vi "2D barcode scanning no PSD 2 scanners.vi"() -> ()   [LabVIEW 2017]
panel:
  out "Horizontal Mirror Driving Angle 1":dynamicdata(graph)
  out "Horizontal Angle Vs. Photodiode Falling 2":cluster{"X":dbl[], "Y":dbl[]}[](graph) caption="XY Graph"
  out "Horizontal Mirror Angle 2":dbl[](graph)
  out "Horizontal Mirror Driving Angle 2":dynamicdata(graph)
  out "Photodiode 2":dynamicdata(graph)
  out "Photodiode 1":dynamicdata(graph)
  in  "All points":bool
  out "Vertical Mirror Angle":dynamicdata(graph)
  out "Horizontal Mirror Angle 1":dynamicdata(graph)
  out "Vertical Angle vs. Photodiode":cluster{"Y":dbl[], "Y":dbl[]}[](graph)
  out "Horizontal Angle vs. Photodiode Falling  1":cluster{"Y":dbl[], "Y":dbl[]}[](graph)
  out "Horizontal Mirror Driving Voltage (common)":dynamicdata(graph)
  out "Vertical Mirror Driving Voltage":dynamicdata(graph)
  in  "stop (F)":bool
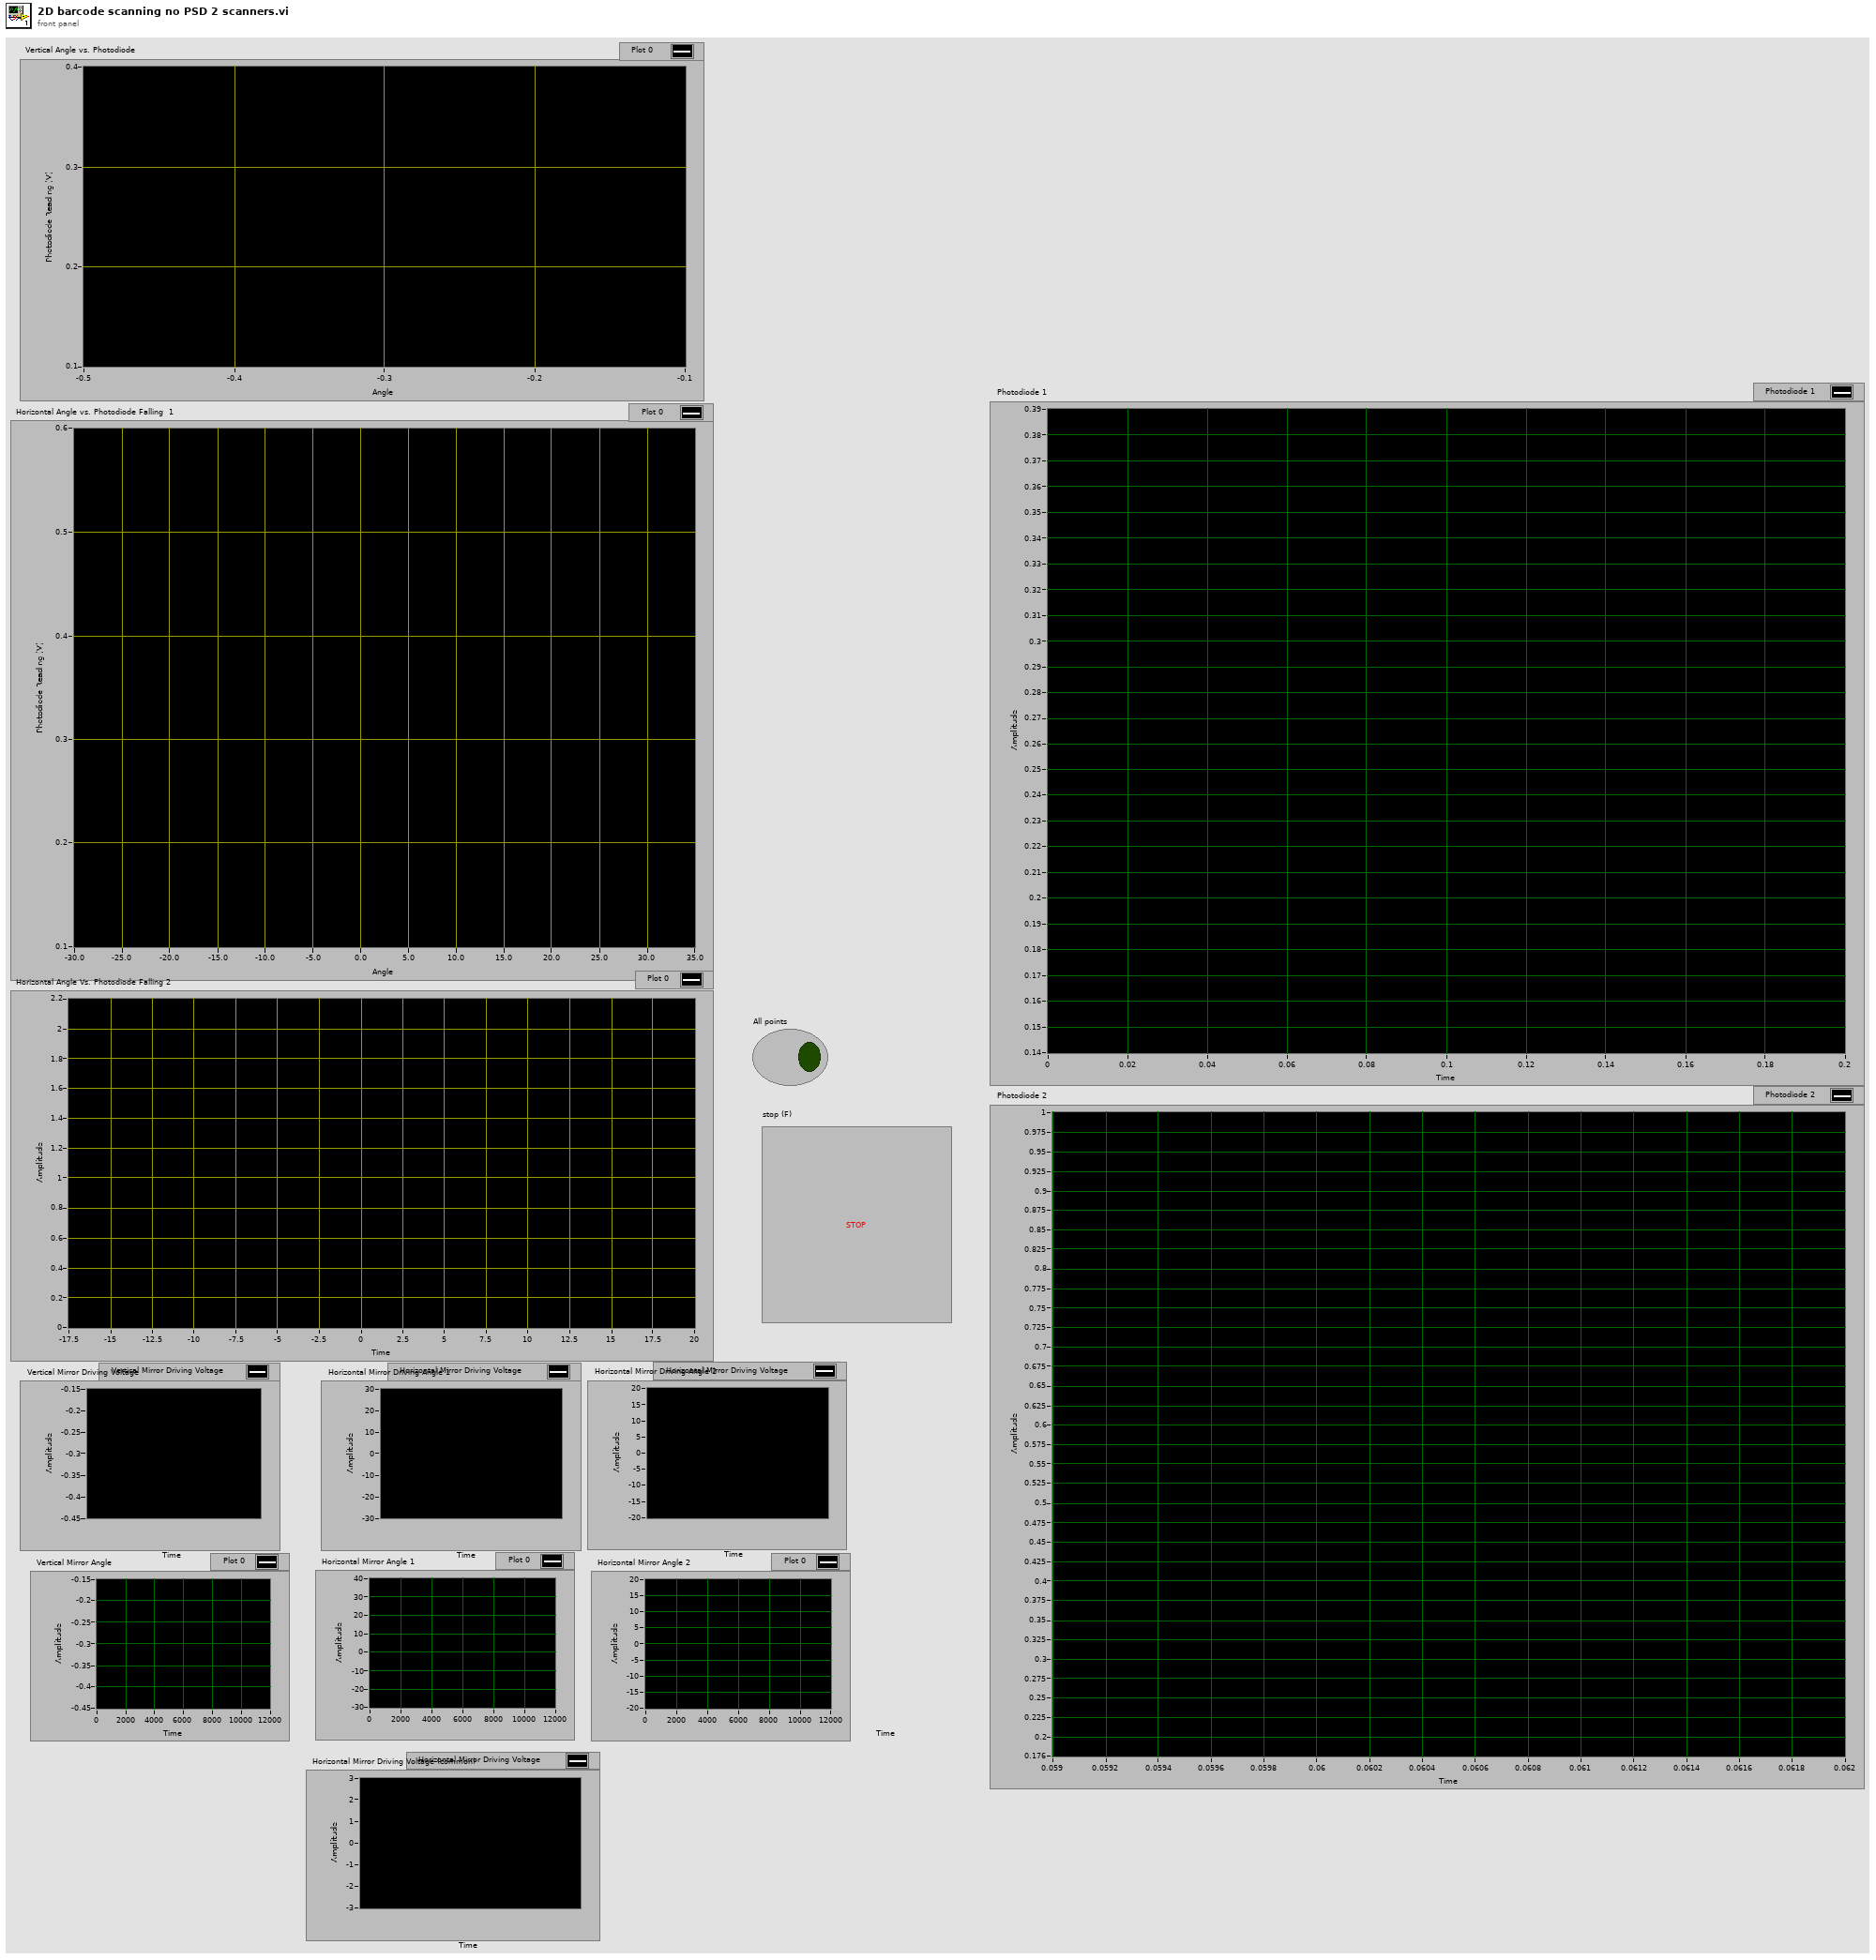
[diagram p1: front panel]
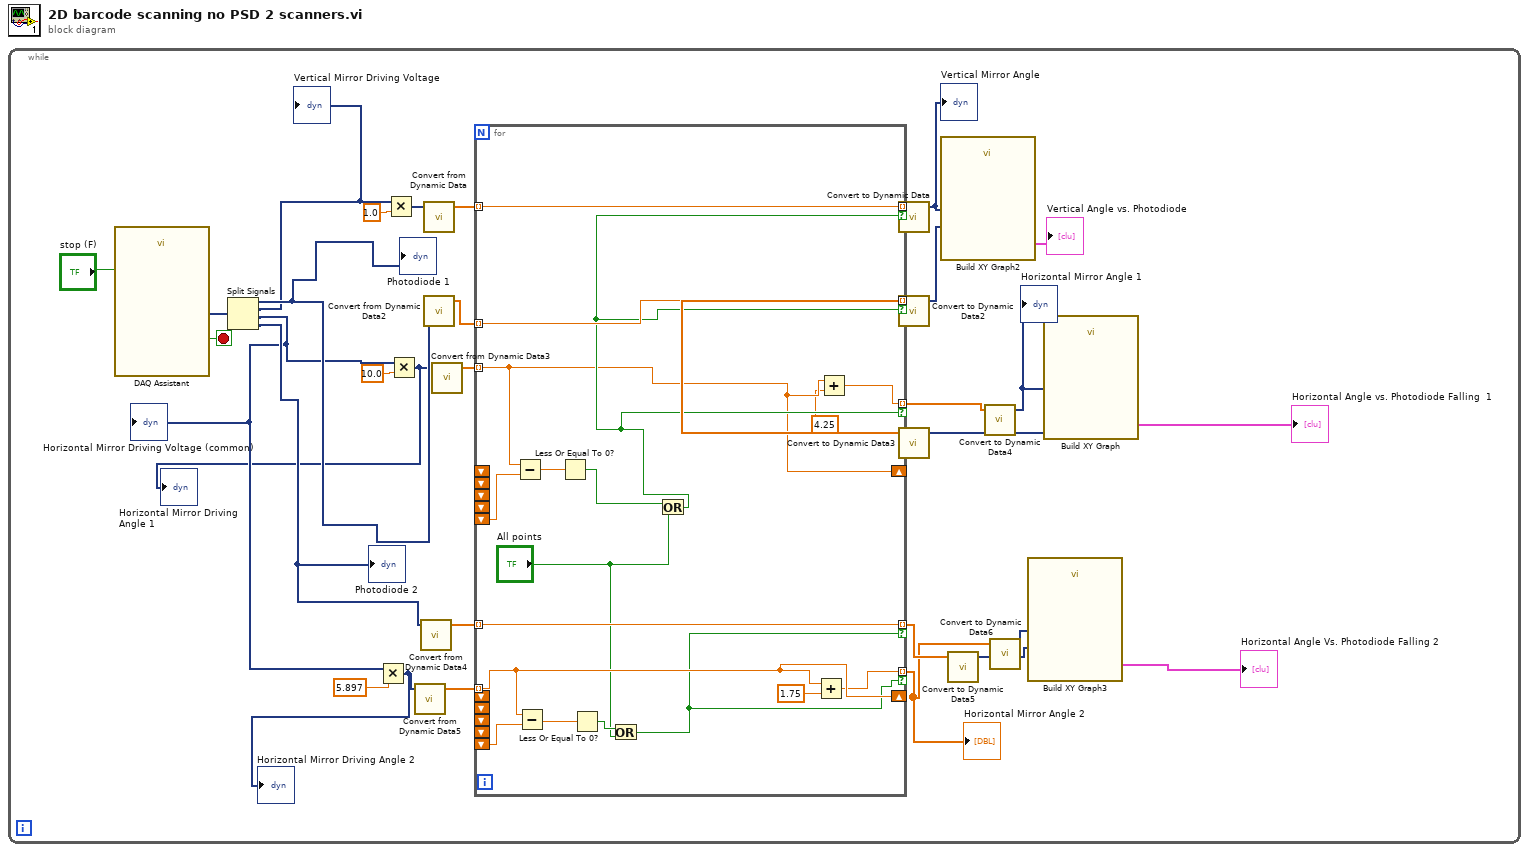
[diagram p0: block diagram]
diagram:
  n1 = while {
    stop <- w31 stop-if-true
    n2 = call "DAQ Assistant"("stop (F)"="stop (F)") -> ("data"=w30:dynamicdata, "stopped"=w31:bool)  [unwired: 15 in, 2 out]
    n3 = Split Signals(w30) -> (w14:dynamicdata, w5:dynamicdata, w3:dynamicdata, w4:dynamicdata)  [unwired: 4 in]
    "Vertical Mirror Driving Voltage" <- w5
    "Horizontal Mirror Driving Voltage (common)" <- w3
    "Photodiode 1" <- w14
    "Photodiode 2" <- w4
    n4 = Multiply(x=w3, y=5.897) -> (x*y=w2:dynamicdata)
    "Horizontal Mirror Driving Angle 2" <- w2
    n5 = Multiply(x=w5, y=1.0) -> (x*y=w24:dynamicdata)
    n6 = Multiply(x=w3, y=10.0) -> (x*y=w1:dynamicdata)
    "Horizontal Mirror Driving Angle 1" <- w1
    n7 = call "Convert from Dynamic Data5"("Dynamic Data Type"=w2) -> ("Array"=w9:dbl[])  [unwired: 3 in]
    n8 = call "Convert from Dynamic Data4"("Dynamic Data Type"=w4) -> ("Array"=w13:dbl[])  [unwired: 3 in]
    n9 = call "Convert from Dynamic Data"("Dynamic Data Type"=w24) -> ("Array"=w23:dbl[])  [unwired: 3 in]
    n10 = call "Convert from Dynamic Data2"("Dynamic Data Type"=w14) -> ("Array"=w22:dbl[])  [unwired: 3 in]
    n11 = call "Convert from Dynamic Data3"("Dynamic Data Type"=w1) -> ("Array"=w18:dbl[])  [unwired: 3 in]
    n12 = for {
      tunnel: [w50] -> w25 mode=indexing if=w47
      tunnel: w23 -> [w50] mode=indexing
      tunnel: w22 -> [w48] mode=indexing
      tunnel: [w48] -> w17 mode=indexing if=w47
      tunnel: w18 -> [w45] mode=indexing
      tunnel: [w44] -> w15 mode=indexing if=w47
      shift-right: [w45] -> _
      shift-left: _ -> [_]
      shift-left: _ -> [_]
      shift-left: _ -> [_]
      shift-left: _ -> [_]
      shift-left: _ -> [w42]
      tunnel: w13 -> [w41] mode=indexing
      tunnel: [w41] -> w12 mode=indexing if=w33
      tunnel: w9 -> [w39] mode=indexing
      shift-right: [w39] -> _
      shift-left: _ -> [_]
      shift-left: _ -> [_]
      shift-left: _ -> [_]
      shift-left: _ -> [_]
      shift-left: _ -> [w34]
      tunnel: [w35] -> w8 mode=indexing if=w33
      n13 = Subtract(x=w45, y=w42) -> (x-y=w49:dbl)
      n14 = Subtract(x=w39, y=w34) -> (x-y=w38:dbl)
      n15 = Less Or Equal To 0?(x=w49) -> (x <= 0?=w46:bool)
      n16 = Less Or Equal To 0?(x=w38) -> (x <= 0?=w37:bool)
      n17 = Or(x=w37, y="All points") -> (x .or. y?=w33:bool)
      n18 = Or(x=w46, y="All points") -> (x .or. y?=w47:bool)
      n19 = Add(x=w39, y=1.75) -> (x+y=w35:dbl)
      n20 = Add(x=w45, y=4.25) -> (x+y=w44:dbl)
    }
    "Horizontal Mirror Angle 2" <- w8
    n21 = call "Convert to Dynamic Data"("Array"=w25) -> ("Dynamic Data Type"=w20:dynamicdata)  [unwired: 3 in]
    "Vertical Mirror Angle" <- w20
    n22 = call "Convert to Dynamic Data2"("Array"=w17) -> ("Dynamic Data Type"=w21:dynamicdata)  [unwired: 3 in]
    n23 = call "Convert to Dynamic Data3"("Array"=w17) -> ("Dynamic Data Type"=w16:dynamicdata)  [unwired: 3 in]
    n24 = call "Build XY Graph2"("Y Input"=w21, "X Input"=w20) -> ("XY Graph"=→"Vertical Angle vs. Photodiode":cluster{"X":dbl[], "Y":dbl[]}[])  [unwired: 8 in, 1 out]
    n25 = call "Convert to Dynamic Data5"("Array"=w12) -> ("Dynamic Data Type"=w11:dynamicdata)  [unwired: 3 in]
    n26 = call "Convert to Dynamic Data4"("Array"=w15) -> ("Dynamic Data Type"=w19:dynamicdata)  [unwired: 3 in]
    "Horizontal Mirror Angle 1" <- w19
    n27 = call "Convert to Dynamic Data6"("Array"=w8) -> ("Dynamic Data Type"=w7:dynamicdata)  [unwired: 3 in]
    n28 = call "Build XY Graph3"("Y Input"=w11, "X Input"=w7) -> ("XY Graph"=→"Horizontal Angle Vs. Photodiode Falling 2":cluster{"X":dbl[], "Y":dbl[]}[])  [unwired: 8 in, 1 out]
    n29 = call "Build XY Graph"("Y Input"=w16, "X Input"=w19) -> ("XY Graph"=→"Horizontal Angle vs. Photodiode Falling  1":cluster{"X":dbl[], "Y":dbl[]}[])  [unwired: 8 in, 1 out]
  }
